vi "Show Reference.vi"(1 "Lower Voltage Threshold Reference":dbl, 2 "Upper Voltage Threshold Reference":dbl, 3 "Show Channel":bool, 4 "Samples per Channel":i32) -> (0 "Reference Levels":dbl[][](array[numeric]))   [LabVIEW 2009]
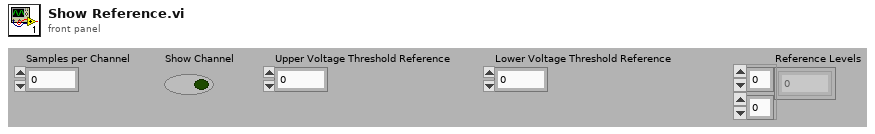
[diagram p1: front panel]
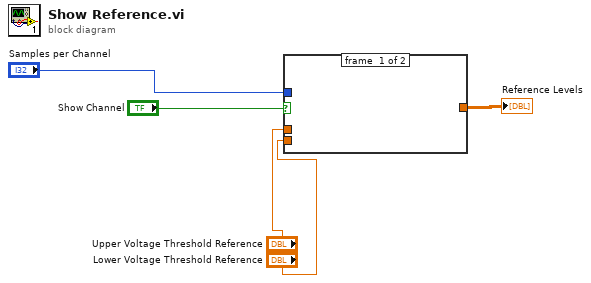
[diagram p0: block diagram]
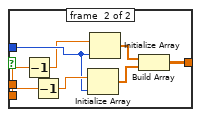
[diagram p2: hidden frame]
diagram:
  n1 = case shown="True" "Show Channel" {
    tunnel: "Samples per Channel" -> [_ w10]
    tunnel: "Upper Voltage Threshold Reference" -> [_ w13]
    tunnel: "Lower Voltage Threshold Reference" -> [_ w12]
    tunnel: [_ w6] -> w5
    frame #0 {
    }
    frame #1 {
      n2 = Decrement(x=w13) -> (x-1=w9:dbl)
      n3 = Decrement(x=w12) -> (x-1=w11:dbl)
      n4 = Initialize Array(w11, w10) -> (w7:dbl[])
      n5 = Initialize Array(w9, w10) -> (w8:dbl[])
      n6 = Build Array(w8, w7) -> (w6:dbl[][])
    }
  }
  "Reference Levels" <- w5
